vi "EEI EXP12.vi"() -> ()   [LabVIEW 2020]
uses:
  <vilib>/numeric/Random Number (Range) U64.vi
  <vilib>/numeric/sub_Random U32.vi
  <vilib>/Utility/file.llb/Write Delimited Spreadsheet (string).vi
panel:
  out "appended array":string[][](array[string])
  in  "Path":path
  in  "Numeric":i32
  out "current time":timestamp
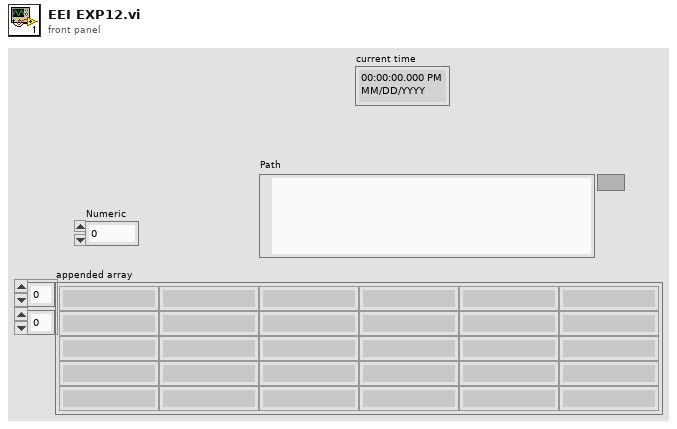
[diagram p1: front panel]
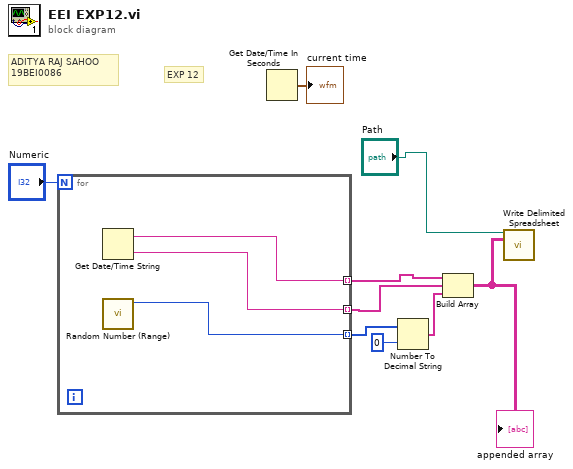
[diagram p0: block diagram]
diagram:
  # "EXP 12"
  # "ADITYA RAJ SAHOO\n19BEI0086"
  n1 = for {
    N: "Numeric" -> [_]
    tunnel: [w12] -> w7 mode=indexing
    tunnel: [w11] -> w6 mode=indexing
    tunnel: [w10] -> w5 mode=indexing
    n2 = Get Date/Time String() -> (date string=w12:string, time string=w11:string)  [unwired: 3 in]
    n3 = call-poly <vilib>:"Random Number (Range).vi"() -> ("number"=w10:u64)  [unwired: 11 in]
  }
  n4 = Get Date/Time In Seconds() -> (seconds since 1Jan1904=→"current time":timestamp)
  n5 = Number To Decimal String(number=w5, width (-)=i16 0) -> (decimal integer string=w2:string[])
  n6 = Build Array(w7, w6, w2) -> (w1:string[][])
  "appended array" <- w1
  n7 = call-poly <vilib>:"Write Delimited Spreadsheet.vi"("file path (dialog if empty)"="Path", "2D data"=w1) -> ()  [unwired: 12 in, 2 out]
